vi "Load Configuration.vi"(8 "error in (no error)":errorcluster, 11 "Client Config in":refnum<class "Client Config.lvclass">) -> (0 "error out":errorcluster, 3 "Client Config out":refnum<class "Client Config.lvclass">)   [LabVIEW 2016]
uses:
  <vilib>/Utility/config.llb/NI_LVConfig.lvlib
  <userlib>/Configuration Dialog Actor/Configuration.lvclass
  Client Config.lvclass
  <vilib>/Utility/config.llb/Write Key (String).vi
  <vilib>/Utility/config.llb/Read Key (U32).vi
  <vilib>/Utility/config.llb/Write Key (U32).vi
  <vilib>/Utility/config.llb/Read Key (String).vi
  \\Mac\Home/Documents/MAL-Framework/user.lib/Common Components/Msmt Configuration/Controller Configuration.lvclass
  C:/Program Files (x86)/National Instruments/LabVIEW 2016/user.lib/Configuration Dialog Actor/Configuration.lvclass
  C:/Program Files (x86)/National Instruments/LabVIEW 2016/vi.lib/ActorFramework/Actor/Actor.lvclass
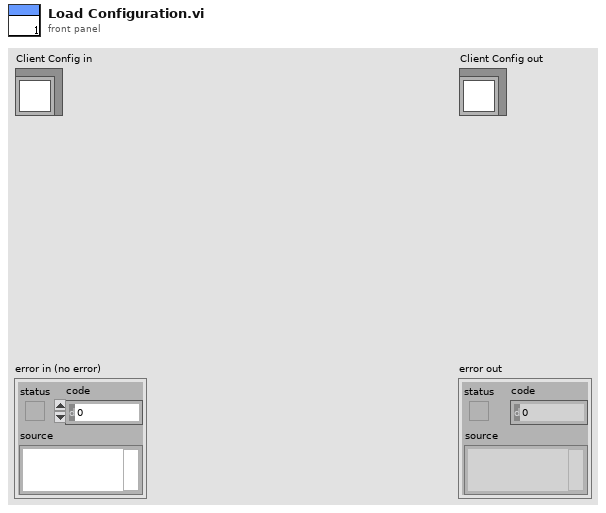
[diagram p1: front panel]
types:
  T1 = typedef "NI_LVConfig.lvlib/Config Data RefNum.ctl" = refnum<k1>
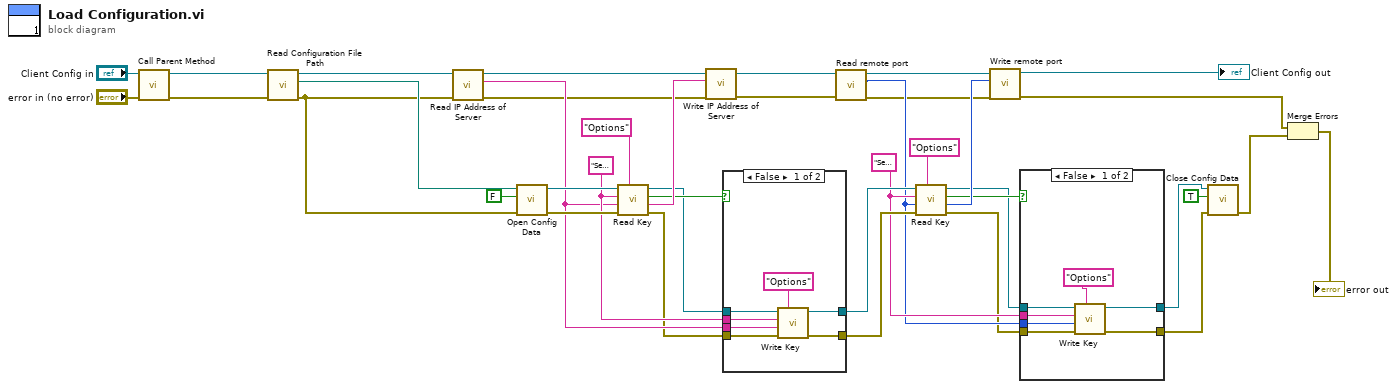
[diagram p0: block diagram]
diagram:
  w11 = "ServerPort" ("key")
  w21 = "ServerIP" ("key")
  n1 = call-parent "Call Parent Method"("error in (no error)"="error in (no error)", "Controller Configuration in"="Client Config in") -> ("error out"=w26:errorcluster, "Controller Configuration out"=w34:refnum<class "Client Config.lvclass">)  [unwired: 8 in]
  n2 = call <userlib>:"Read Configuration File Path.vi"("error in (no error)"=w26, "Configuration in"=w34) -> ("error out"=w7:errorcluster, "Configuration File Path"=w33:path, "Configuration out"=w30:refnum<class "Client Config.lvclass">)  [unwired: 7 in]
  n3 = call "Read IP Address of Server.vi"("error in (no error)"=w7, "Client Config in"=w30) -> ("error out"=w6:errorcluster, "IP Address of Server"=w20:string, "Client Config out"=w31:refnum<class "Client Config.lvclass">)  [unwired: 7 in]
  n4 = call <vilib>:"Open Config Data.vi"("error in (no error)"=w7, "create file if necessary (T)"=FALSE, "configuration file path"=w33) -> ("error out"=w35:errorcluster, "refnum"=w36:T1)  [unwired: 6 in, 1 out]
  n5 = call-poly <vilib>:"Read Key.vi"("section"="Options", "error in (no error)"=w35, "default value"=w20, "key"=w21, "refnum"=w36) -> ("error out"=w17:errorcluster, "value"=w24:string, "found?"=w23:bool, "refnum out"=w22:T1)  [unwired: 3 in]
  n6 = call "Write IP Address of Server.vi"("error in (no error)"=w6, "IP Address of Server"=w24, "Client Config in"=w31) -> ("error out"=w5:errorcluster, "Client Config out"=w29:refnum<class "Client Config.lvclass">)  [unwired: 7 in]
  n7 = case shown="False" w23 {
    tunnel: w22 -> [w46 w47]
    tunnel: w21 -> [w45 _]
    tunnel: w20 -> [w44 _]
    tunnel: [w43 w48] -> w18
    tunnel: w17 -> [w42 w48]
    tunnel: [w41 w47] -> w16
    frame False {
      n8 = call-poly <vilib>:"Write Key.vi"("section"="Options", "error in (no error)"=w42, "value"=w44, "key"=w45, "refnum"=w46) -> ("error out"=w43:errorcluster, "refnum out"=w41:T1)  [unwired: 4 in, 1 out]
    }
    frame True {
    }
  }
  n9 = call "Read remote port.vi"("error in (no error)"=w5, "Client Config in"=w29) -> ("error out"=w4:errorcluster, "remote port"=w10:u16, "Client Config out"=w28:refnum<class "Client Config.lvclass">)  [unwired: 7 in]
  n10 = call-poly <vilib>:"Read Key.vi"("section"="Options", "error in (no error)"=w18, "default value"=w10, "key"=w11, "refnum"=w16) -> ("error out"=w9:errorcluster, "value"=w25:u32, "found?"=w15:bool, "refnum out"=w14:T1)  [unwired: 3 in]
  n11 = call "Write remote port.vi"("error in (no error)"=w4, "remote port"=w25, "Client Config in"=w28) -> ("error out"=w3:errorcluster, "Client Config out"=→"Client Config out":refnum<class "Client Config.lvclass">)  [unwired: 7 in]
  n12 = case shown="False" w15 {
    tunnel: w14 -> [w55 w57]
    tunnel: [w54 w57] -> w13
    tunnel: w11 -> [w53 _]
    tunnel: w10 -> [w52 _]
    tunnel: w9 -> [w51 w56]
    tunnel: [w50 w56] -> w8
    frame False {
      n13 = call-poly <vilib>:"Write Key.vi"("section"="Options", "error in (no error)"=w51, "value"=w52, "key"=w53, "refnum"=w55) -> ("error out"=w50:errorcluster, "refnum out"=w54:T1)  [unwired: 4 in, 1 out]
    }
    frame True {
    }
  }
  n14 = call <vilib>:"Close Config Data.vi"("error in (no error)"=w8, "write file if changed (T)"=TRUE, "refnum"=w13) -> ("error out"=w2:errorcluster)  [unwired: 7 in, 1 out]
  n15 = Merge Errors(w3, w2) -> (→"error out":errorcluster)
